vi "filtro_ecg_adaptativo.vi"() -> ()   [LabVIEW 2014]
uses:
  <vilib>/Analysis/baseanly.llb/Real Dot Product.vi
  <vilib>/Analysis/NI_AALBase.lvlib
  <vilib>/Analysis/NI_AALPro.lvlib
panel:
  out "o_s":dbl[](graph)
  out "o_e":dbl[](graph)
  out "w":dbl[](array[numeric])
  out "delay":dbl[](array[numeric])
  in  "beta":dbl
  out "o_e":dbl[](array[numeric])
  out "o_s":dbl[](array[numeric])
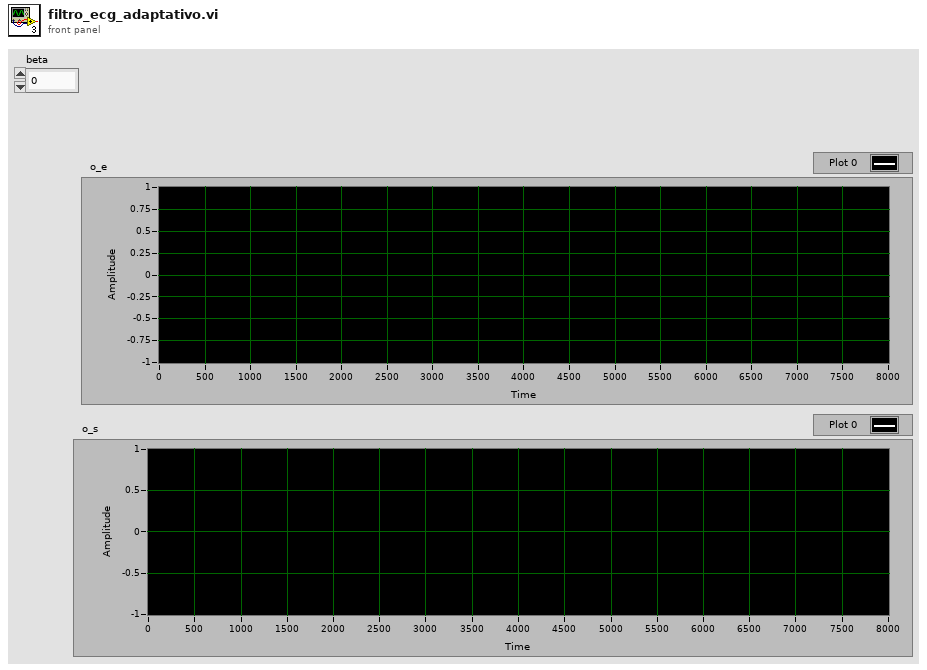
[diagram p1: front panel]
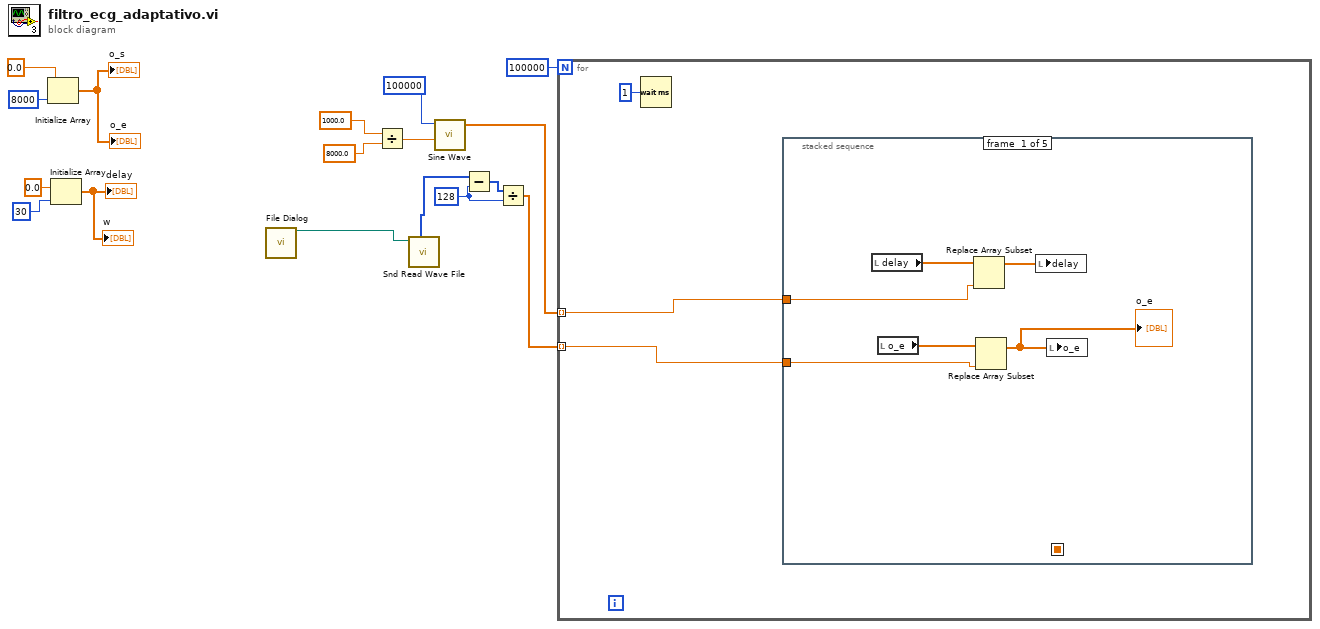
[diagram p0: block diagram]
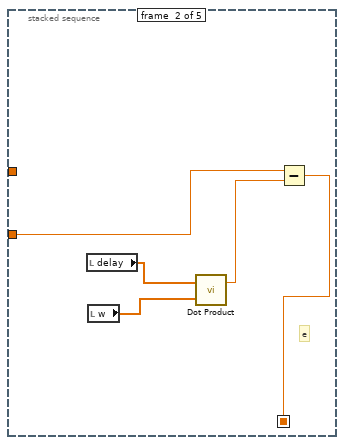
[diagram p2: hidden frame]
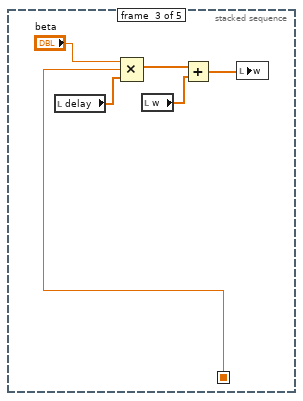
[diagram p3: hidden frame]
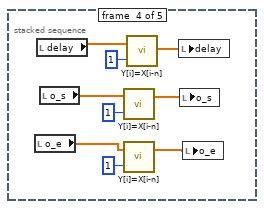
[diagram p4: hidden frame]
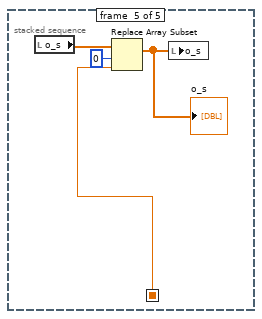
[diagram p5: hidden frame]
diagram:
  w2 = 128
  n1 = Initialize Array(0.0 ("element"), 8000 ("dimension size")) -> (→"o_s" →"o_e":dbl[])
  n2 = Initialize Array(0.0 ("element"), 30 ("dimension size")) -> (→"delay" →"w":dbl[])
  n3 = call "File Dialog"() -> ("selected path"=w13:path)  [unwired: 12 in, 3 out]
  n4 = Divide(x=1000.0, y=8000.0) -> (x/y=w16:dbl)
  n5 = call <vilib>:"Snd Read Wave File.vi"("wave file path"=w13) -> ("mono 8-bit"=w5:u8[])  [unwired: 4 in, 6 out]
  n6 = call <vilib>:"Sine Wave.vi"("samples"=100000, "frequency"=w16) -> ("sine wave"=w4:dbl[])  [unwired: 3 in, 2 out]
  n7 = Subtract(x=w5, y=w2) -> (x-y=w3:i32[])
  n8 = Divide(x=w3, y=w2) -> (x/y=w1:dbl[])
  n9 = for {
    N: 100000 -> [_]
    tunnel: w4 -> [w20] mode=indexing
    tunnel: w1 -> [w19] mode=indexing
    n10 = Wait (ms)(milliseconds to wait=u32 1) -> ()  [unwired: 1 out]
    n11 = stacked-sequence {
      seq-local: [_ w29 _ _ _] -> [_ _ w36 _ w49]
      tunnel: w20 -> [w26 _ _ _ _]
      tunnel: w19 -> [w22 w28 _ _ _]
      frame #0 {
        n12 = local read "delay"() -> (w25:dbl[])
        n13 = local read "o_e"() -> (w23:dbl[])
        n14 = Replace Array Subset(array=w25, new element=w26) -> (w24:dbl[])  [unwired: 1 in]
        n15 = Replace Array Subset(array=w23, new element=w22) -> (w21:dbl[])  [unwired: 1 in]
        "o_e" <- w21
        n16 = local write "delay"(w24) -> ()
        n17 = local write "o_e"(w21) -> ()
      }
      frame #1 {
        # "e"
        n18 = local read "delay"() -> (w31:dbl[])
        n19 = local read "w"() -> (w30:dbl[])
        n20 = call-poly <vilib>:"Dot Product.vi"("Y Vector"=w30, "X Vector"=w31) -> ("X * Y"=w27:dbl)  [unwired: 1 out]
        n21 = Subtract(x=w28, y=w27) -> (x-y=w29:dbl)
      }
      frame #2 {
        n22 = local read "delay"() -> (w35:dbl[])
        n23 = Compound Arithmetic op=MULTIPLY("beta", w36, w35) -> (w34:dbl[])
        n24 = local read "w"() -> (w33:dbl[])
        n25 = Add(x=w34, y=w33) -> (x+y=w32:dbl[])
        n26 = local write "w"(w32) -> ()
      }
      frame #3 {
        n27 = local read "o_e"() -> (w39:dbl[])
        n28 = local read "delay"() -> (w46:dbl[])
        n29 = local read "o_s"() -> (w42:dbl[])
        n30 = call <vilib>:"Y[i]=X[i-n].vi"("shifts: n"=1, "Input Array"=w42) -> ("Shifted Array"=w41:dbl[])  [unwired: 1 out]
        n31 = call <vilib>:"Y[i]=X[i-n].vi"("shifts: n"=1, "Input Array"=w39) -> ("Shifted Array"=w38:dbl[])  [unwired: 1 out]
        n32 = call <vilib>:"Y[i]=X[i-n].vi"("shifts: n"=1, "Input Array"=w46) -> ("Shifted Array"=w44:dbl[])  [unwired: 1 out]
        n33 = local write "delay"(w44) -> ()
        n34 = local write "o_s"(w41) -> ()
        n35 = local write "o_e"(w38) -> ()
      }
      frame #4 {
        n36 = local read "o_s"() -> (w50:dbl[])
        n37 = Replace Array Subset(array=w50, new element=w49, index=0) -> (w47:dbl[])
        "o_s" <- w47
        n38 = local write "o_s"(w47) -> ()
      }
    }
  }
